vi "Power Preserve Sign.vi"() -> ()   [LabVIEW 2012]
panel:
  out "Out":dbl
  in  "Number":dbl
  in  "Power":dbl
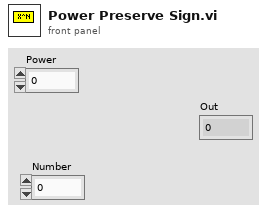
[diagram p1: front panel]
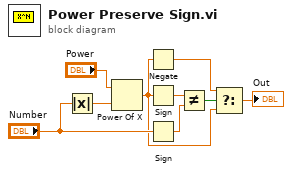
[diagram p0: block diagram]
diagram:
  n1 = Absolute Value(x="Number") -> (abs(x)=w7:dbl)
  n2 = Power Of X(1:w7, 2:"Power") -> (0:w4:dbl)
  n3 = Negate(x=w4) -> (-x=w6:dbl)
  n4 = Sign(1:w4) -> (0:w2:dbl)
  n5 = Sign(1:"Number") -> (0:w3:dbl)
  n6 = Not Equal?(x=w2, y=w3) -> (x != y?=w1:bool)
  n7 = Select(t=w6, s=w1, f=w4) -> (s? t:f=→"Out":dbl)
